vi "Rosliny.vi"() -> ()   [LabVIEW 2023]
uses:
  Rosliny_zmienne.vi
panel:
  in  "Ustaw":bool
  in  "Ilosc zraszaczy":dbl
  in  "Rok":dbl
  in  "Miesiac":dbl
  in  "Dzien":dbl
  in  "Minuta":dbl
  in  "Godzina":dbl
  in  "Sekcja tryb reczny":dbl
  in  "Czas podlewania":dbl
  in  "Liczba sekcji":dbl=1.0
  in  "Podlewaj tryb reczny":bool
  in  "Podlewaj":bool
  # "Harmonogram"
  # "Automatyczny"
  # "Reczny"
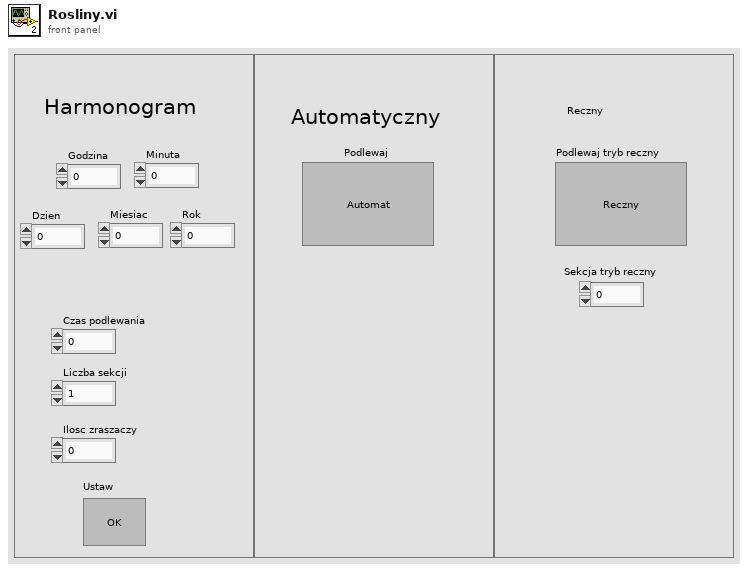
[diagram p1: front panel]
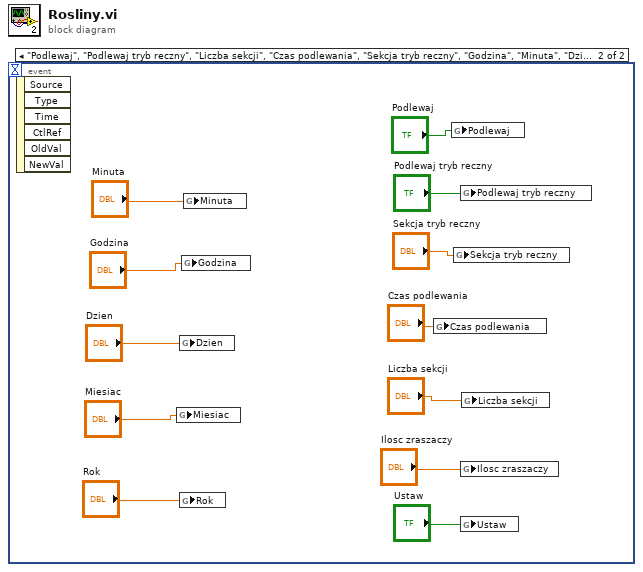
[diagram p0: block diagram]
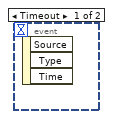
[diagram p2: hidden frame]
diagram:
  n1 = event shown="[1] \"Podlewaj\", \"Podlewaj tryb reczny\", \"Liczba sekcji\", \"Czas podlewania\", \"Sekcja tryb reczny\", \"Godzina\", \"Minuta\", \"Dzien\", \"Miesiac\", \"Rok\", \"Ilosc zraszaczy\": Value Change" {
    selector: _ -> [_ _]
    dyn-events: _ -> [_ _]
    timeout: _ -> [_ _]
    event Timeout {
      n2 = event-data() -> ()  [unwired: 1 in, 3 out]
    }
    event "Podlewaj", "Podlewaj tryb reczny", "Liczba sekcji", "Czas podlewania", "Sekcja tryb reczny", "Godzina", "Minuta", "Dzien", "Miesiac", "Rok", "Ilosc zraszaczy": Value Change {
      n3 = event-data() -> ()  [unwired: 1 in, 6 out]
      n4 = global write "Rosliny_zmienne.vi" "Miesiac"("Miesiac") -> ()
      n5 = global write "Rosliny_zmienne.vi" "Dzien"("Dzien") -> ()
      n6 = global write "Rosliny_zmienne.vi" "Rok"("Rok") -> ()
      n7 = global write "Rosliny_zmienne.vi" "Godzina"("Godzina") -> ()
      n8 = global write "Rosliny_zmienne.vi" "Minuta"("Minuta") -> ()
      n9 = global write "Rosliny_zmienne.vi" "Czas podlewania"("Czas podlewania") -> ()
      n10 = global write "Rosliny_zmienne.vi" "Podlewaj"("Podlewaj") -> ()
      n11 = global write "Rosliny_zmienne.vi" "Sekcja tryb reczny"("Sekcja tryb reczny") -> ()
      n12 = global write "Rosliny_zmienne.vi" "Podlewaj tryb reczny"("Podlewaj tryb reczny") -> ()
      n13 = global write "Rosliny_zmienne.vi" "Ilosc zraszaczy"("Ilosc zraszaczy") -> ()
      n14 = global write "Rosliny_zmienne.vi" "Ustaw"("Ustaw") -> ()
      n15 = global write "Rosliny_zmienne.vi" "Liczba sekcji"("Liczba sekcji") -> ()
    }
  }
